vi "CPP_GaussianPeakPlugIn.vi"() -> (5 "Plug in titles":string[](array[string]), 7 "Plug in values":string[](array[string]))   [LabVIEW 2011]
uses:
  Globals/Meas_global.vi
  Utilities/gaussianFit/GaussianGlobal.vi
panel:
  out "RakeSpacing":dbl
  in  "PositionAllowance(mm)":dbl=50.0
  out "FitSDwithin(Factor)OfPrediction?":bool
  out "bigEnough?":bool
  out "closeEnough?":bool
  in  "AmplitudeTolerance (%)":dbl=5.0
  in  "LocationTolerance":dbl=0.1 caption="LocationTolerance(*predictedSD)"
  in  "FitvsPredictionSDFactor":dbl=2.5
  out "ConcentrationData":dbl[](array[numeric])
  out "PositionData":dbl[](array[numeric])
  out "FitStatus":string
  out "FitResidual":dbl
  out "FitStdDev":dbl
  out "FitMax":dbl
  out "FitCenter":dbl
  out "XY Graph":T1(graph)
  # "!! 5-hole 1-5 must be connected to Channels 1-5 !!"
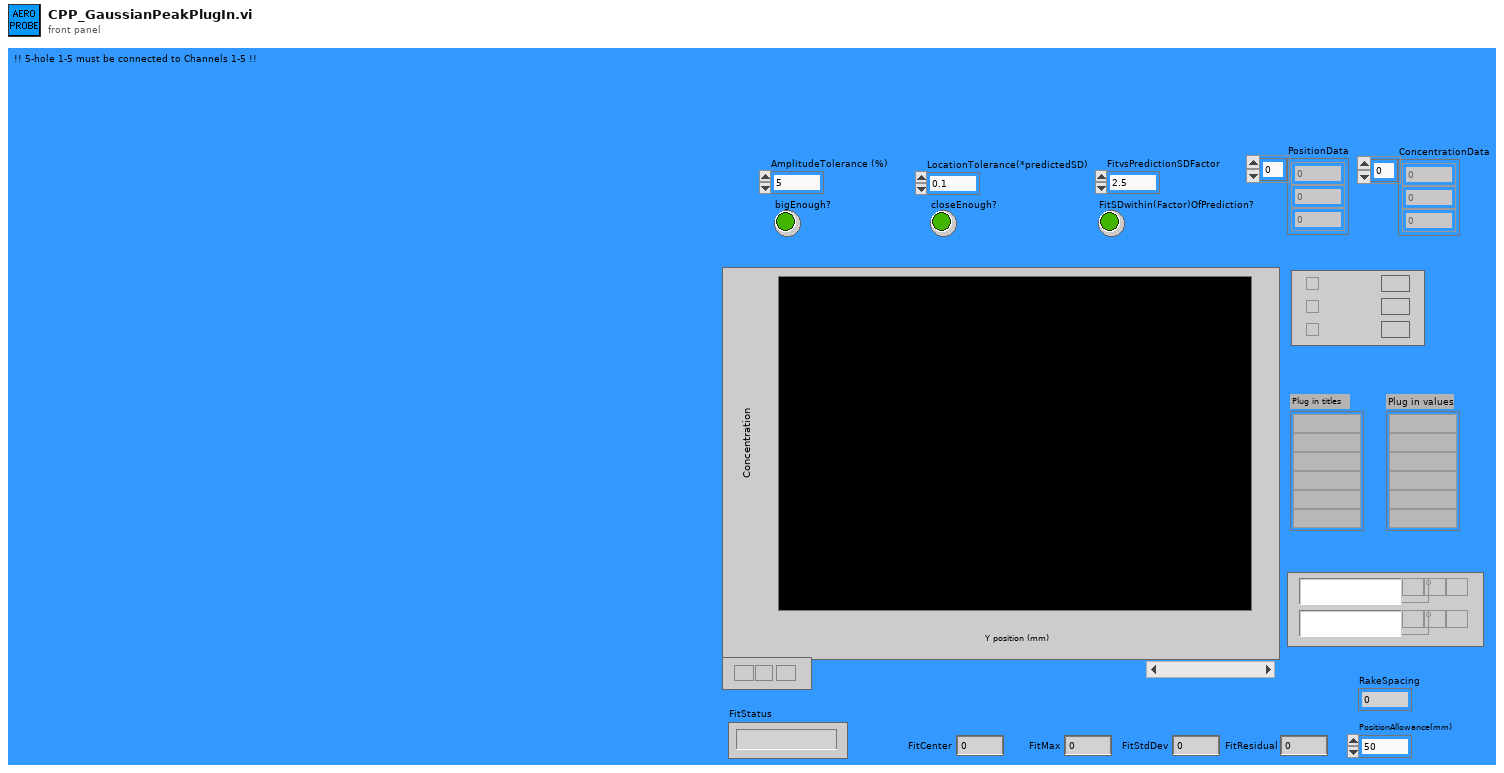
[diagram p1: front panel]
types:
  T1 = cluster{"Array - Numeric":dbl[], "Array - Numeric":dbl[]}[]
  T2 = typedef "Analysis_info_cluster.ctl" = cluster{"Colour":u32, "Inst type":T3, "Inst name":string, "Symbol":string, "Code name":string, "Extra Info":string, "Inst Array":T4, "Extra Titles":string[], "Extra Values":string[], "Eng Values":dbl[], "Time (ms)":dbl[], "Voltage":dbl[], "U":dbl, "u^2":dbl, "u^3":dbl, "u^4":dbl, "Skew_u":dbl, "Kurt_u":dbl, "Sd Error in Mean":dbl, "% u'/U":dbl, "X":dbl, "Y":dbl, "Z":dbl, "Spectra":T5, "Autocorrelation":T5, "Timescale integral to 25%":dbl, "Sd Error in Variance":dbl, "Calib File":path, "Calib Constants":dbl[], "Histogram":T5, "Output Position":bool, "Full Stats":bool, "Weighting":dbl[], "Av Sampling Rate":dbl, "Av No of Samples":dbl, "Total Meas Time (s)":dbl}
  T3 = typedef "Inst_type.ctl" = enum16{"Propeller anemometer", "Raw voltage", "Pressure Transducer", "Pitot-static tube", "Preston tube", "Hot wire", "Cross wire 1", "Cross wire 2", "Generic Linear", "Generic Polynomial", "Generic BackPoly", "Fast FID", "Thermocouple", "Cold wire", "Pulsed Wire", "LDA Vel", "LDA Tran time", "LDA Arr time"}
  T4 = typedef "Instrument_Array.ctl" = enum16{"PWA", "LDA", "Analogue"}
  T5 = typedef "XY_Plot_Cluster.ctl" = cluster{"First Name":string, "Second Name":string, "X axis name":string, "Y axis name":string, "X array":dbl[], "Y array":dbl[]}
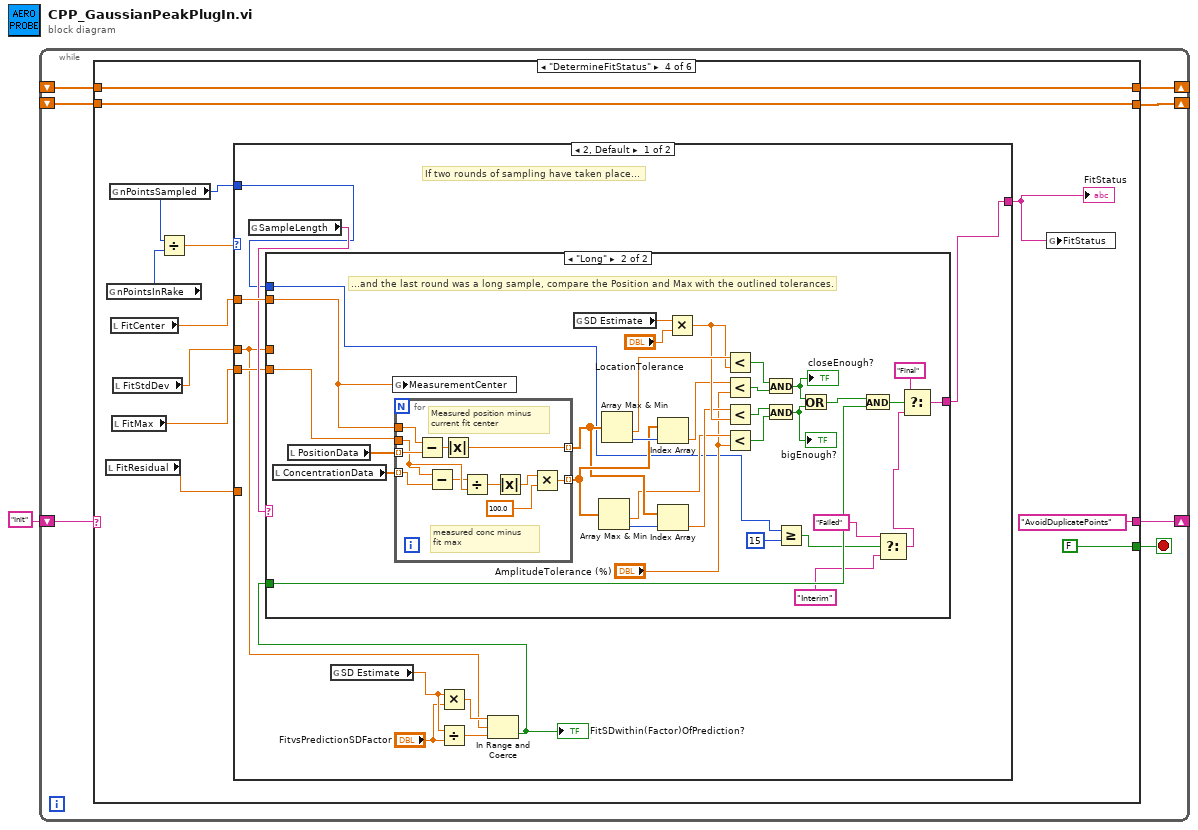
[diagram p0: block diagram]
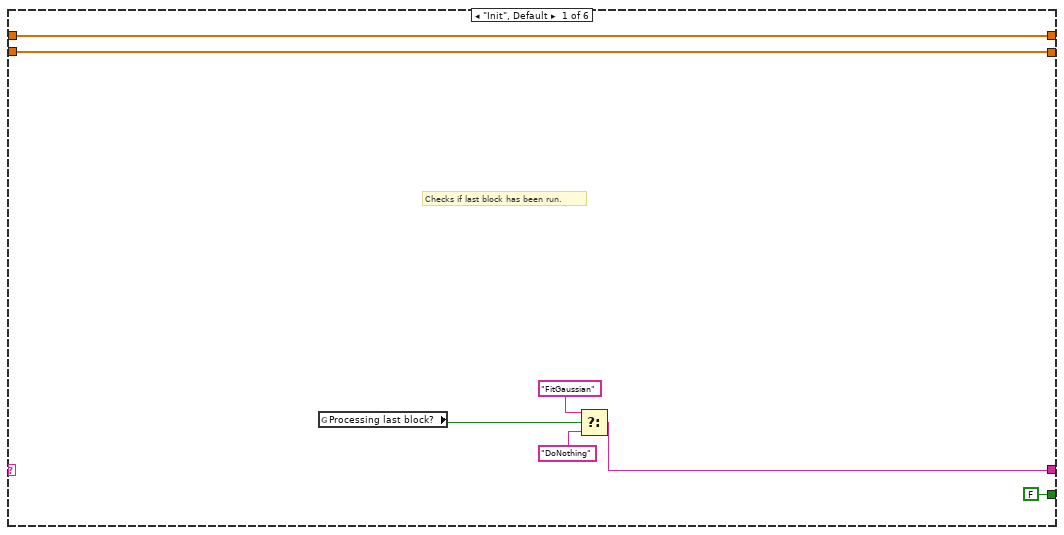
[diagram p2: hidden frame]
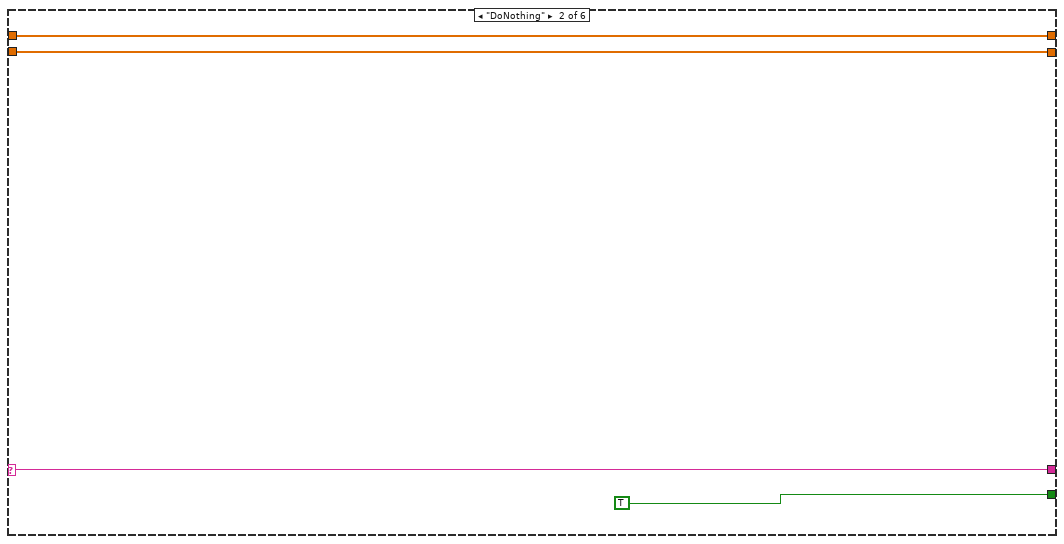
[diagram p3: hidden frame]
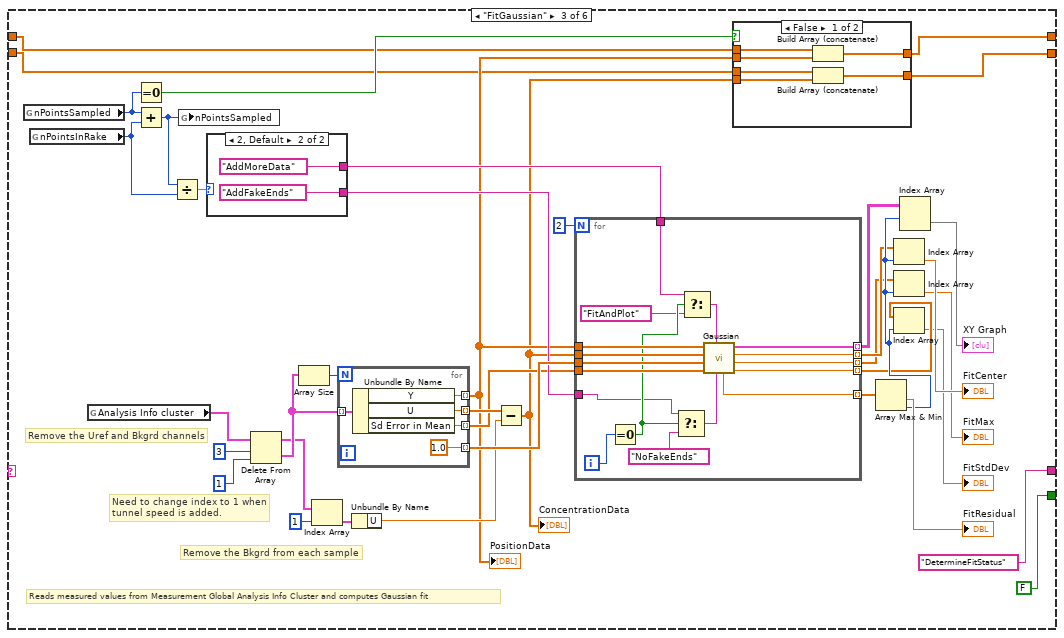
[diagram p4: hidden frame]
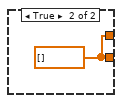
[diagram p5: hidden frame]
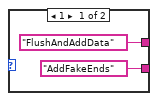
[diagram p6: hidden frame]
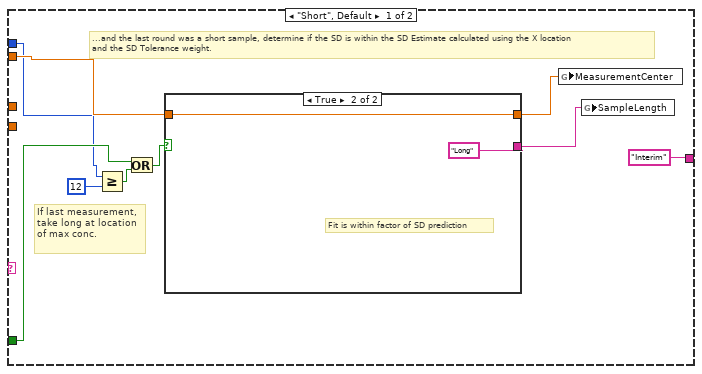
[diagram p7: hidden frame]
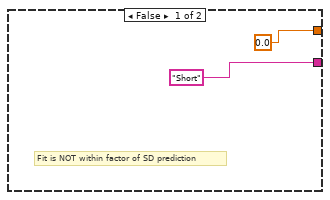
[diagram p8: hidden frame]
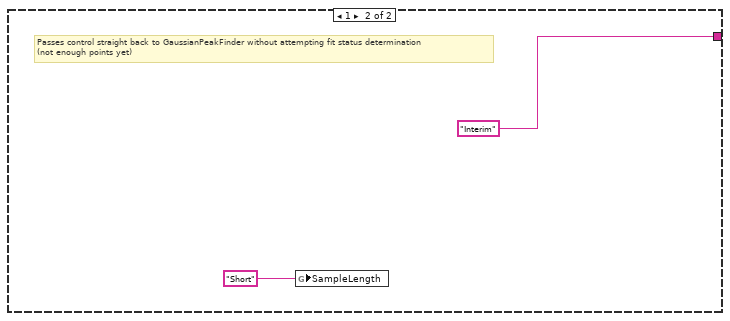
[diagram p9: hidden frame]
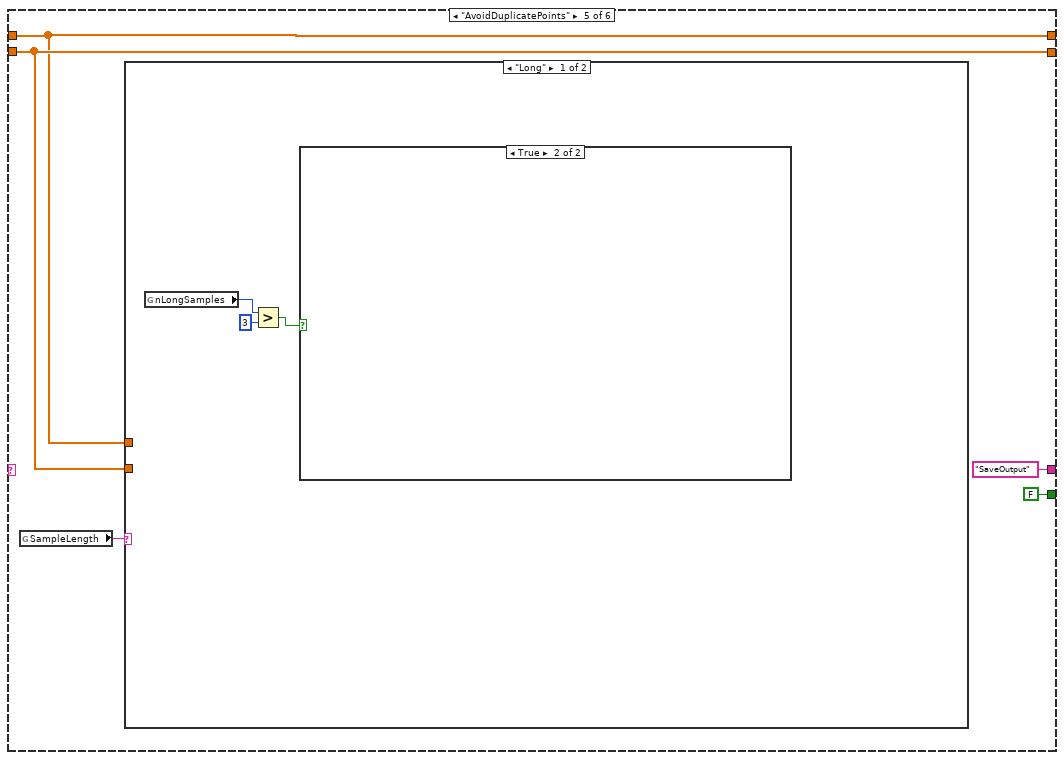
[diagram p10: hidden frame]
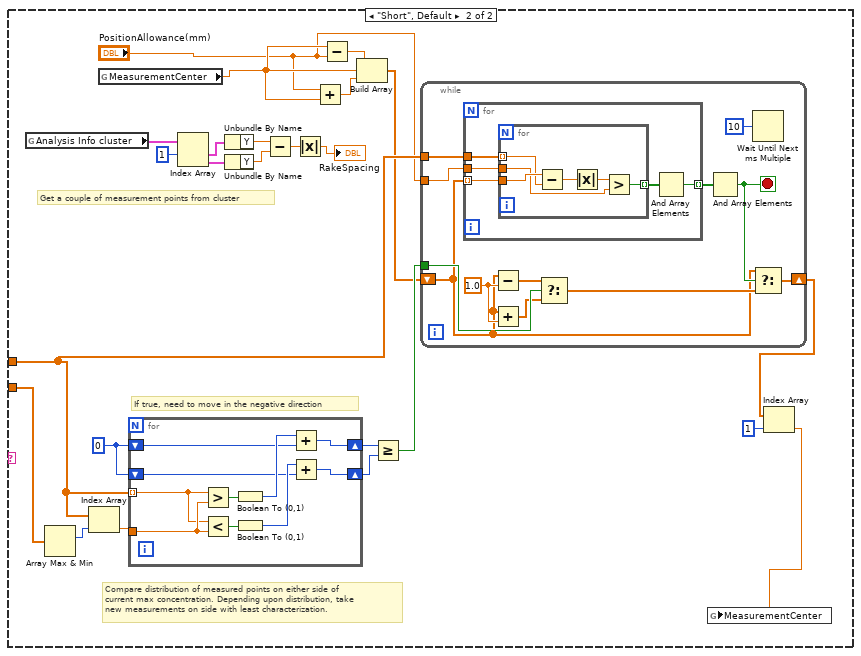
[diagram p12: hidden frame]
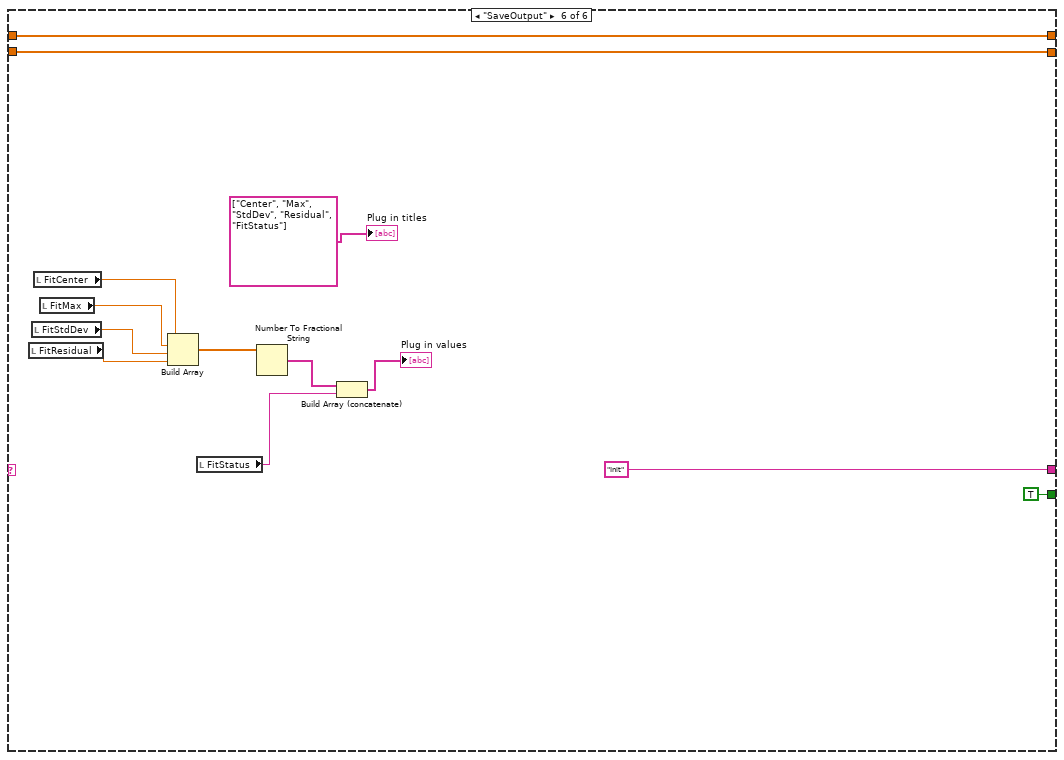
[diagram p13: hidden frame]
diagram:
  n1 = while {
    shift-right: [w7] -> _
    shift-left: "Init" -> [w8]
    shift-right: [w5] -> _
    shift-left: _ -> [w4]
    shift-right: [w3] -> _
    shift-left: _ -> [w2]
    stop <- w6 stop-if-true
    n2 = case shown="\"DetermineFitStatus\"" w8 {
      selector: w8 -> [_ w19 _ _ _ _]
      tunnel: [w15 w19 "DetermineFitStatus" ("f") "AvoidDuplicatePoints" "SaveOutput" ("f") "Init"] -> w7
      tunnel: [FALSE TRUE FALSE FALSE FALSE TRUE] -> w6
      tunnel: [w10 w17 w37 w92 w175 w240] -> w5
      tunnel: w4 -> [w10 w17 w39 w92 w175 w240]
      tunnel: [w9 w16 w36 w93 w176 w239] -> w3
      tunnel: w2 -> [w9 w16 w35 w93 w176 w239]
      frame "Init", Default {
        # "Checks if last block has been run."
        n3 = global read "Meas_global.vi" "Processing last block?"() -> (w14:bool)
        n4 = Select(t="FitGaussian", s=w14, f="DoNothing") -> (s? t:f=w15:string)
      }
      frame "DoNothing" {
      }
      frame "FitGaussian" {
        # "Need to change index to 1 when\ntunnel speed is added."
        # "Remove the Bkgrd from each sample"
        # "Remove the Uref and Bkgrd channels"
        # "Reads measured values from Measurement Global Analysis Info Cluster and computes Gaussian fit"
        n5 = global read "GaussianGlobal.vi" "nPointsSampled"() -> (w33:i32)
        n6 = global read "GaussianGlobal.vi" "nPointsInRake"() -> (w53:i32)
        n7 = global read "Meas_global.vi" "Analysis Info cluster"() -> (w51:T2[])
        n8 = Equal To 0?(x=w33) -> (x = 0?=w40:bool)
        n9 = Add(x=w33, y=w53) -> (x+y=w32:i32)
        n10 = Divide(x=w32, y=w53) -> (x/y=w56:dbl)
        n11 = global write "GaussianGlobal.vi" "nPointsSampled"(w32) -> ()
        n12 = case shown="2, Default" w56 {
          tunnel: ["FlushAndAddData" ("Mode") "AddMoreData" ("Mode")] -> w55
          tunnel: ["AddFakeEnds" ("Combo Box") "AddFakeEnds" ("Combo Box")] -> w54
          frame 1 {
          }
          frame 2, Default {
          }
        }
        n13 = Delete From Array(array=w51, length=3, index=1) -> (deleted portion=w48:T2[], array with subset deleted=w47:T2[])
        n14 = Array Size(array=w48) -> (size(s)=w49:i32)
        n15 = Index Array(array=w47, index=1) -> (element=w46:T2)
        n16 = for {
          N: w49 -> [_]
          tunnel: w48 -> [w87] mode=indexing
          tunnel: [w91] -> w38 mode=indexing
          tunnel: [w90] -> w42 mode=indexing
          tunnel: [w89] -> w41 mode=indexing
          tunnel: [1.0] -> w58 mode=indexing
          n17 = Unbundle By Name(w87) -> ("Y"=w91:dbl, "U"=w90:dbl, "Sd Error in Mean"=w89:dbl)
        }
        "PositionData" <- w38
        n18 = Unbundle By Name(w46) -> ("U"=w45:dbl)
        n19 = Subtract(x=w42, y=w45) -> (x-y=w34:dbl[])
        "ConcentrationData" <- w34
        n20 = for {
          N: 2 -> [_]
          tunnel: w58 -> [w75]
          tunnel: [w74] -> w28 mode=indexing
          tunnel: [w73] -> w26 mode=indexing
          tunnel: [w72] -> w25 mode=indexing
          tunnel: [w71] -> w24 mode=indexing
          tunnel: [w70] -> w31 mode=indexing
          tunnel: w55 -> [w64]
          tunnel: w54 -> [w62]
          tunnel: w41 -> [w69]
          tunnel: w38 -> [w68]
          tunnel: w34 -> [w67]
          i -> [w66]
          n21 = Equal To 0?(x=w66) -> (x = 0?=w65:bool)
          n22 = Select(t=w62, s=w65, f="NoFakeEnds" ("Combo Box")) -> (s? t:f=w61:string)
          n23 = Select(t=w64, s=w65, f="FitAndPlot" ("Mode")) -> (s? t:f=w63:string)
          n24 = call "Gaussian.vi"("Fake Ends?"=w61, "Mode"=w63, "YerrorIn"=w69, "XerrorIn"=w75, "YdataIn"=w67, "XdataIn"=w68) -> ("StdDev"=w71:dbl, "Max"=w72:dbl, "Center"=w73:dbl, "XY Graph"=w74:T1, "residual"=w70:dbl)  [unwired: 1 in]
        }
        n25 = case shown="False" w40 {
          tunnel: w38 -> [w81 _]
          tunnel: [w79 w82] -> w37
          tunnel: w39 -> [w80 _]
          tunnel: [w76 w82] -> w36
          tunnel: w35 -> [w78 _]
          tunnel: w34 -> [w77 _]
          frame False {
            n26 = Build Array (concatenate)(w80, w81) -> (w79:dbl[])
            n27 = Build Array (concatenate)(w78, w77) -> (w76:dbl[])
          }
          frame True {
            w82 = dbl[] []
          }
        }
        n28 = Array Max & Min(array=w31) -> (min value=→"FitResidual":dbl, min index (indices)=w29:i32)  [unwired: 2 out]
        n29 = Index Array(array=w26, index=w29) -> (element=→"FitCenter":dbl)
        n30 = Index Array(array=w25, index=w29) -> (element=→"FitMax":dbl)
        n31 = Index Array(array=w24, index=w29) -> (element=→"FitStdDev":dbl)
        n32 = Index Array(array=w28, index (row)=w29) -> (element=→"XY Graph":T1)  [unwired: 1 in]
      }
      frame "DetermineFitStatus" {
        n33 = local read "FitResidual"() -> (w97:dbl)
        n34 = global read "GaussianGlobal.vi" "nPointsInRake"() -> (w102:i32)
        n35 = global read "GaussianGlobal.vi" "nPointsSampled"() -> (w94:i32)
        n36 = local read "FitCenter"() -> (w98:dbl)
        n37 = local read "FitMax"() -> (w99:dbl)
        n38 = local read "FitStdDev"() -> (w100:dbl)
        n39 = Divide(x=w94, y=w102) -> (x/y=w101:dbl)
        n40 = case shown="2, Default" w101 {
          tunnel: w100 -> [w105 _]
          tunnel: w99 -> [w107 _]
          tunnel: w98 -> [w114 _]
          tunnel: w97 -> [_ _]
          tunnel: [w104 "Interim"] -> w95
          tunnel: w94 -> [w106 _]
          frame 2, Default {
            # "If two rounds of sampling have taken place..."
            n41 = global read "GaussianGlobal.vi" "SampleLength"() -> (w113:string)
            n42 = global read "GaussianGlobal.vi" "SD Estimate"() -> (w111:dbl)
            n43 = Multiply(x=w111, y="FitvsPredictionSDFactor") -> (x*y=w109:dbl)
            n44 = Divide(x=w111, y="FitvsPredictionSDFactor") -> (x/y=w112:dbl)
            n45 = In Range and Coerce(upper limit=w109, x=w105, lower limit=w112) -> (In Range?=w108:bool)  [unwired: 1 out]
            "FitSDwithin(Factor)OfPrediction?" <- w108
            n46 = case shown="\"Long\"" w113 {
              tunnel: w114 -> [w121 w137]
              tunnel: w107 -> [_ w160]
              tunnel: ["Interim" w138] -> w104
              tunnel: w105 -> [_ _]
              tunnel: w108 -> [w118 w135]
              tunnel: w106 -> [w115 w130]
              frame "Short", Default {
                # "If last measurement, take long at location of max conc."
                # "...and the last round was a short sample, determine if the SD is within the SD Estimate calculated using the X location\nand the SD Tolerance weight."
                n47 = Greater Or Equal?(x=w115, y=12) -> (x >= y?=w116:bool)
                n48 = Or(x=w118, y=w116) -> (x .or. y?=w117:bool)
                n49 = case shown="True" w117 {
                  tunnel: ["Short" "Long"] -> w122
                  tunnel: w121 -> [_ w126]
                  tunnel: [0.0 ("f") w126] -> w120
                  frame False {
                    # "Fit is NOT within factor of SD prediction"
                  }
                  frame True {
                    # "Fit is within factor of SD prediction"
                  }
                }
                n50 = global write "GaussianGlobal.vi" "MeasurementCenter"(w120) -> ()
                n51 = global write "GaussianGlobal.vi" "SampleLength"(w122) -> ()
              }
              frame "Long" {
                # "...and the last round was a long sample, compare the Position and Max with the outlined tolerances."
                n52 = local read "ConcentrationData"() -> (w159:dbl[])
                n53 = local read "PositionData"() -> (w158:dbl[])
                n54 = global write "GaussianGlobal.vi" "MeasurementCenter"(w137) -> ()
                n55 = for {
                  tunnel: w158 -> [w171] mode=indexing
                  tunnel: w159 -> [w170] mode=indexing
                  tunnel: w137 -> [w169]
                  tunnel: w160 -> [w168]
                  tunnel: [w163] -> w156 mode=indexing
                  tunnel: [w161] -> w154 mode=indexing
                  # "measured conc minus \nfit max"
                  # "Measured position minus\ncurrent fit center"
                  n56 = Subtract(x=w169, y=w171) -> (x-y=w162:dbl)
                  n57 = Subtract(x=w168, y=w170) -> (x-y=w167:dbl)
                  n58 = Absolute Value(x=w162) -> (abs(x)=w161:dbl)
                  n59 = Divide(x=w167, y=w168) -> (x/y=w166:dbl)
                  n60 = Absolute Value(x=w166) -> (abs(x)=w164:dbl)
                  n61 = Multiply(x=w164, y=100.0) -> (x*y=w163:dbl)
                }
                n62 = global read "GaussianGlobal.vi" "SD Estimate"() -> (w151:dbl)
                n63 = Array Max & Min(array=w156) -> (min value=w147:dbl, min index (indices)=w155:i32)  [unwired: 2 out]
                n64 = Array Max & Min(array=w154) -> (min value=w153:dbl, min index (indices)=w157:i32)  [unwired: 2 out]
                n65 = Index Array(array=w156, index=w157) -> (element=w149:dbl)
                n66 = Index Array(array=w154, index=w155) -> (element=w148:dbl)
                n67 = Multiply(x=w151, y="LocationTolerance") -> (x*y=w150:dbl)
                n68 = Less?(x=w153, y=w150) -> (x < y?=w145:bool)
                n69 = Less?(x=w149, y="AmplitudeTolerance (%)") -> (x < y?=w144:bool)
                n70 = Less?(x=w148, y=w150) -> (x < y?=w143:bool)
                n71 = Less?(x=w147, y="AmplitudeTolerance (%)") -> (x < y?=w142:bool)
                n72 = And(x=w145, y=w144) -> (x .and. y?=w141:bool)
                "closeEnough?" <- w141
                n73 = And(x=w143, y=w142) -> (x .and. y?=w140:bool)
                "bigEnough?" <- w140
                n74 = Greater Or Equal?(x=w130, y=15) -> (x >= y?=w132:bool)
                n75 = Or(x=w141, y=w140) -> (x .or. y?=w136:bool)
                n76 = And(x=w136, y=w135) -> (x .and. y?=w134:bool)
                n77 = Select(t="Failed", s=w132, f="Interim") -> (s? t:f=w128:string)
                n78 = Select(t="Final", s=w134, f=w128) -> (s? t:f=w138:string)
              }
            }
          }
          frame 1 {
            # "Passes control straight back to GaussianPeakFinder without attempting fit status determination\n(not enough points yet)"
            n79 = global write "GaussianGlobal.vi" "SampleLength"("Short" ("SampleLength")) -> ()
          }
        }
        "FitStatus" <- w95
        n80 = global write "GaussianGlobal.vi" "FitStatus"(w95) -> ()
      }
      frame "AvoidDuplicatePoints" {
        n81 = global read "GaussianGlobal.vi" "SampleLength"() -> (w174:string)
        n82 = case shown="\"Long\"" w174 {
          tunnel: w176 -> [_ w205]
          tunnel: w175 -> [_ w188]
          frame "Long" {
            n83 = global read "GaussianGlobal.vi" "nLongSamples"() -> (w181:i32)
            n84 = Greater?(x=w181, y=3) -> (0:w179:bool)
            n85 = case shown="True" w179 {
              frame False {
              }
              frame True {
              }
            }
          }
          frame "Short", Default {
            w202 = i16 0
            # "Get a couple of measurement points from cluster"
            # "If true, need to move in the negative direction"
            # "Compare distribution of measured points on either side of\ncurrent max concentration. Depending upon distribution, take\nnew measurements on side with least characterization."
            n86 = global read "Meas_global.vi" "Analysis Info cluster"() -> (w199:T2[])
            n87 = Array Max & Min(array=w205) -> (max index (indices)=w204:i32)  [unwired: 3 out]
            n88 = Index Array(array=w188, index=w204) -> (element=w203:dbl)
            n89 = global read "GaussianGlobal.vi" "MeasurementCenter"() -> (w189:dbl)
            n90 = for {
              tunnel: w203 -> [w238]
              tunnel: w188 -> [w237] mode=indexing
              shift-right: [w232] -> w201
              shift-left: w202 -> [w231]
              shift-right: [w230] -> w200
              shift-left: w202 -> [w229]
              n91 = Greater?(x=w237, y=w238) -> (0:w236:bool)
              n92 = Less?(x=w237, y=w238) -> (x < y?=w235:bool)
              n93 = Boolean To (0,1)(Boolean=w236) -> (0, 1=w233:i16)
              n94 = Boolean To (0,1)(Boolean=w235) -> (0, 1=w234:i16)
              n95 = Add(x=w233, y=w231) -> (x+y=w232:i16)
              n96 = Add(x=w234, y=w229) -> (x+y=w230:i16)
            }
            n97 = Index Array(array=w199, index #1=1 ("index")) -> (element #1=w197:T2, element #2=w196:T2)  [unwired: 1 in]
            n98 = Unbundle By Name(w197) -> ("Y"=w195:dbl)
            n99 = Unbundle By Name(w196) -> ("Y"=w194:dbl)
            n100 = Subtract(x=w195, y=w194) -> (x-y=w193:dbl)
            n101 = Absolute Value(x=w193) -> (abs(x)=→"RakeSpacing":dbl)
            n102 = Add(x="PositionAllowance(mm)", y=w189) -> (x+y=w191:dbl)
            n103 = Subtract(x=w189, y="PositionAllowance(mm)") -> (x-y=w190:dbl)
            n104 = Build Array(w190, w189, w191) -> (w185:dbl[])
            n105 = Greater Or Equal?(x=w201, y=w200) -> (x >= y?=w186:bool)
            n106 = while {
              tunnel: w188 -> [w217]
              tunnel: w186 -> [w214]
              tunnel: "PositionAllowance(mm)" -> [w211]
              shift-right: [w207] -> w184
              shift-left: w185 -> [w208]
              stop <- w215 stop-if-true
              w212 = 1.0 ("y")
              n107 = for {
                tunnel: w208 -> [w221] mode=indexing
                tunnel: w217 -> [w222]
                tunnel: w211 -> [w220]
                tunnel: [w218] -> w216 mode=indexing
                n108 = for {
                  tunnel: w222 -> [w227] mode=indexing
                  tunnel: w221 -> [w228]
                  tunnel: w220 -> [w224]
                  tunnel: [w223] -> w219 mode=indexing
                  n109 = Subtract(x=w228, y=w227) -> (x-y=w226:dbl)
                  n110 = Absolute Value(x=w226) -> (abs(x)=w225:dbl)
                  n111 = Greater?(x=w225, y=w224) -> (0:w223:bool)
                }
                n112 = And Array Elements(Boolean array=w219) -> (logical AND=w218:bool)
              }
              n113 = Subtract(x=w208, y=w212) -> (x-y=w213:dbl[])
              n114 = Add(x=w208, y=w212) -> (x+y=w210:dbl[])
              n115 = Select(t=w213, s=w214, f=w210) -> (s? t:f=w209:dbl[])
              n116 = And Array Elements(Boolean array=w216) -> (logical AND=w215:bool)
              n117 = Wait Until Next ms Multiple(millisecond multiple=u32 10) -> ()  [unwired: 1 out]
              n118 = Select(t=w208, s=w215, f=w209) -> (s? t:f=w207:dbl[])
            }
            n119 = Index Array(array=w184, index=1) -> (element=w182:dbl)
            n120 = global write "GaussianGlobal.vi" "MeasurementCenter"(w182) -> ()
          }
        }
      }
      frame "SaveOutput" {
        (unwired) TRUE
        n121 = local read "FitResidual"() -> (w246:dbl)
        n122 = local read "FitStdDev"() -> (w247:dbl)
        n123 = local read "FitCenter"() -> (w249:dbl)
        n124 = local read "FitMax"() -> (w248:dbl)
        n125 = Build Array(w249, w248, w247, w246) -> (w245:dbl[])
        n126 = local read "FitStatus"() -> (w243:string)
        n127 = Number To Fractional String(number=w245) -> (F-format string=w244:string[])  [unwired: 3 in]
        n128 = Build Array (concatenate)(w244, w243) -> (→"Plug in values":string[])
        "Plug in titles" <- string[] ["Center", "Max", "StdDev", "Residual", "FitStatus"] ("Plug in titles")
      }
    }
  }
